vi "getFileFolderName.vi"(6 "regular expression":string="JPG", 8 "Directory":string="d:\\BACKUP", 9 "name or relative path":string, 11 "base path":path) -> (1 "Source":path, 2 "date/time string 2":string, 3 "Destination":path)   [LabVIEW 2012]
panel:
  out "file or folder exists?":bool
  out "x > y?":bool
  out "error out 2":errorcluster
  out "error out":errorcluster
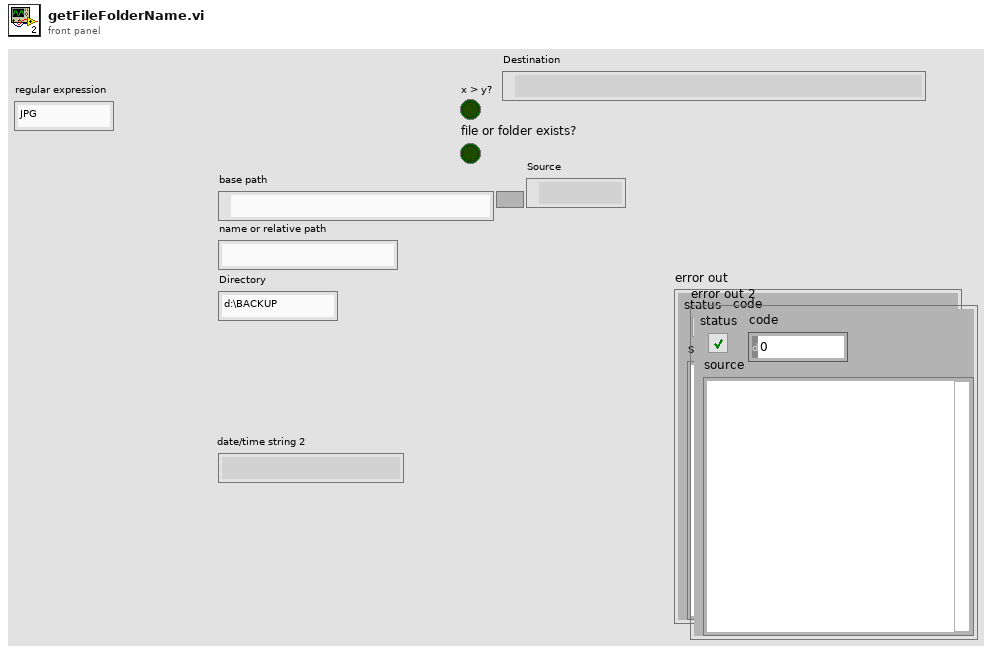
[diagram p1: front panel]
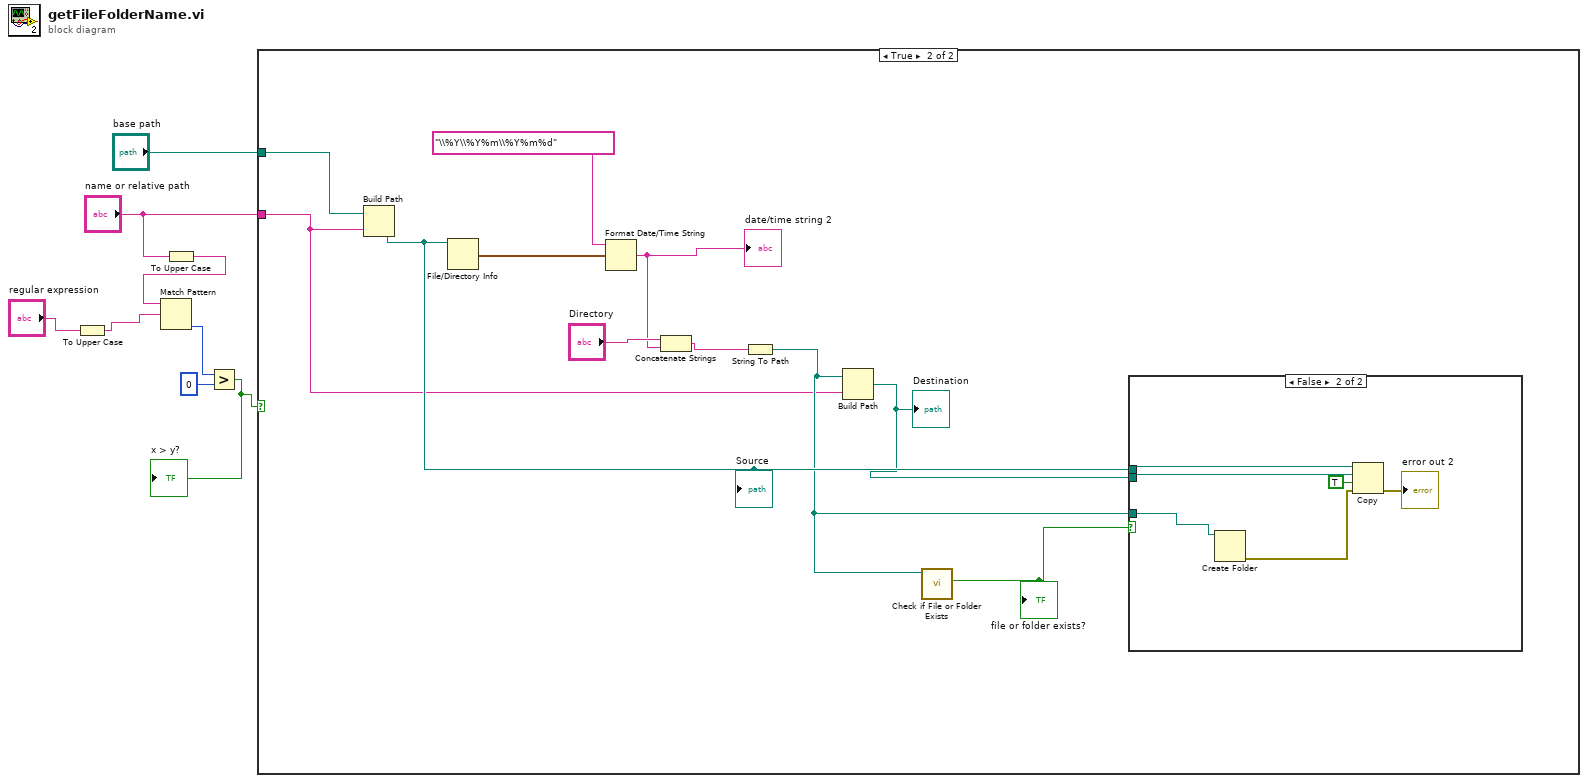
[diagram p0: block diagram]
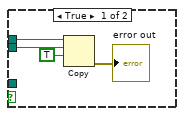
[diagram p3: hidden frame]
diagram:
  n1 = To Upper Case(1:"regular expression") -> (0:w6:string)
  n2 = To Upper Case(1:"name or relative path") -> (0:w1:string)
  n3 = Match Pattern(string=w1, regular expression=w6) -> (offset past match=w5:i32)  [unwired: 1 in, 3 out]
  n4 = Greater?(x=w5, y=0) -> (0:w3:bool)
  "x > y?" <- w3
  n5 = case shown="True" w3 {
    tunnel: "base path" -> [_ w17]
    tunnel: "name or relative path" -> [_ w9]
    frame False {
    }
    frame True {
      n6 = Build Path(base path=w17, name or relative path=w9) -> (appended path=w16:path)
      "Source" <- w16
      n7 = File/Directory Info(path=w16) -> (last mod=w19:timestamp)  [unwired: 1 in, 6 out]
      n8 = Format Date/Time String(time format string (%c)="\\%Y\\%Y%m\\%Y%m%d", seconds (now)=w19) -> (date/time string=w14:string)  [unwired: 1 in]
      "date/time string 2" <- w14
      n9 = Concatenate Strings("Directory", w14) -> (w13:string)
      n10 = String To Path(string=w13) -> (path=w10:path)
      n11 = Build Path(base path=w10, name or relative path=w9) -> (appended path=w12:path)
      "Destination" <- w12
      n12 = call <vilib>:"Check if File or Folder Exists.vi"("path"=w10) -> ("file or folder exists?"=w11:bool)  [unwired: 8 in, 2 out]
      "file or folder exists?" <- w11
      n13 = case shown="False" w11 {
        tunnel: w16 -> [w23 w29]
        tunnel: w12 -> [w20 w26]
        tunnel: w10 -> [_ w25]
        frame True {
          n14 = Copy(9:TRUE ("overwrite (F)"), 10:w20, 11:w23) -> (0:→"error out":errorcluster)  [unwired: 2 in, 2 out]
        }
        frame False {
          n15 = Create Folder(path (use dialog)=w25) -> (error out=w24:errorcluster)  [unwired: 2 in, 2 out]
          n16 = Copy(8:w24, 9:TRUE ("overwrite (F)"), 10:w26, 11:w29) -> (0:→"error out 2":errorcluster)  [unwired: 1 in, 2 out]
        }
      }
    }
  }
